vi "getBGOpenCVIP.vi"(1 "Image":T1) -> (0 "return type":i32)   [LabVIEW 2012]
uses:
  <vilib>/vision/Image Controls.llb/IMAQ Image.ctl
  OpenCvGlobals.vi
  <userlib>/OpenCVImProc/CatWalkLabviewDLLd.dll
  <userlib>/OpenCVImProc/CatWalkLabviewDLL.dll
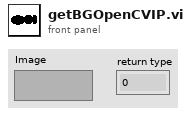
[diagram p1: front panel]
types:
  T1 = typedef "IMAQ Image.ctl" = refnum<image>
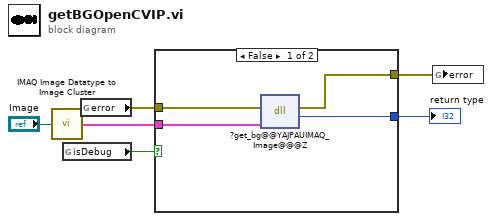
[diagram p0: block diagram]
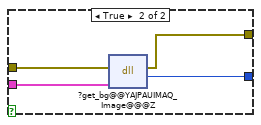
[diagram p2: hidden frame]
diagram:
  n1 = call <vilib>:"IMAQ Image Datatype to Image Cluster.vi"("Image"="Image") -> ("Image (dup)"=w3:cluster{string, u32})
  n2 = global read "OpenCvGlobals.vi" "isDebug"() -> (w6:bool)
  n3 = global read "OpenCvGlobals.vi" "error"() -> (w1:errorcluster)
  n4 = case shown="False" w6 {
    tunnel: [w9 w12] -> w5
    tunnel: [w10 w13] -> w4
    tunnel: w3 -> [w8 w14]
    tunnel: w1 -> [w7 w11]
    frame False {
      n5 = dll-call lib="C:/Program Files (x86)/National Instruments/LabVIEW 2012/user.lib/OpenCVImProc/CatWalkLabviewDLL.dll" fn="?get_bg@@YAJPAUIMAQ_Image@@@Z"(error in=w7, "image"=w8) -> (error out=w10:errorcluster, "return type"=w9:i32)  [unwired: 3 in, 1 out]
    }
    frame True {
      n6 = dll-call lib="C:/Program Files (x86)/National Instruments/LabVIEW 2012/user.lib/OpenCVImProc/CatWalkLabviewDLLd.dll" fn="?get_bg@@YAJPAUIMAQ_Image@@@Z"(error in=w11, "image"=w14) -> (error out=w13:errorcluster, "return type"=w12:i32)  [unwired: 3 in, 1 out]
    }
  }
  "return type" <- w5
  n7 = global write "OpenCvGlobals.vi" "error"(w4) -> ()
